vi "Read.vi"(0 "REF IN":refnum<k24>, 1 "error in":errorcluster, 2 "Path":path, 3 "Begin":bool, 4 "stop":bool, 5 "stop 2":bool, 9 "V":dbl, 11 "A":dbl) -> (14 "new reference 2":refnum<k24>, 15 "error out":errorcluster, 16 "String":string)   [LabVIEW 2017]
uses:
  C:/KMotion434/KMotion/Release/KMotion_dotNet.dll
panel:
  out "lines":string[](array[string])
  out "element":dbl
  out "Status Check Done":dbl format="%11.1f"
  out "Numeric":dbl
  out "Array":string[](array[string])
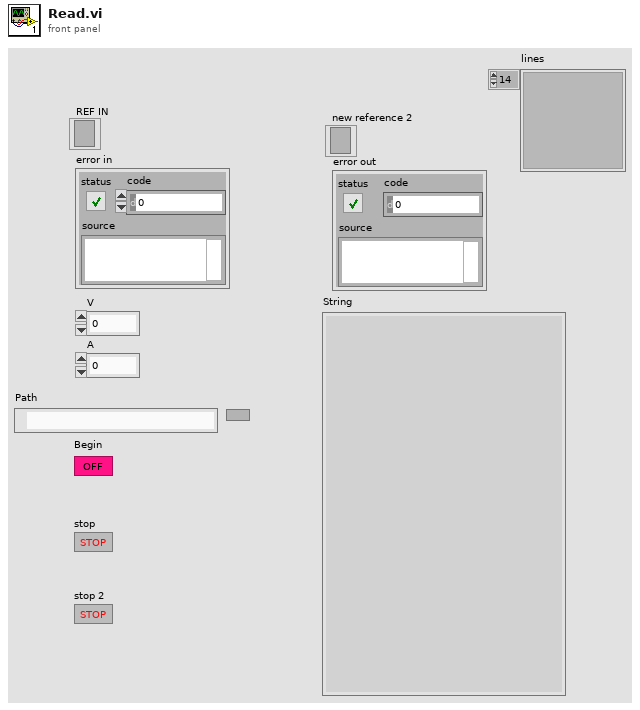
[diagram p1: front panel]
types:
  T1 = cluster{"[0]":dbl, "[1]":dbl, "[2]":dbl, "[3]":dbl, "[4]":dbl, "[5]":dbl, "[6]":dbl, "[7]":dbl, "[8]":dbl, "[9]":dbl, "[10]":dbl, "[11]":dbl}
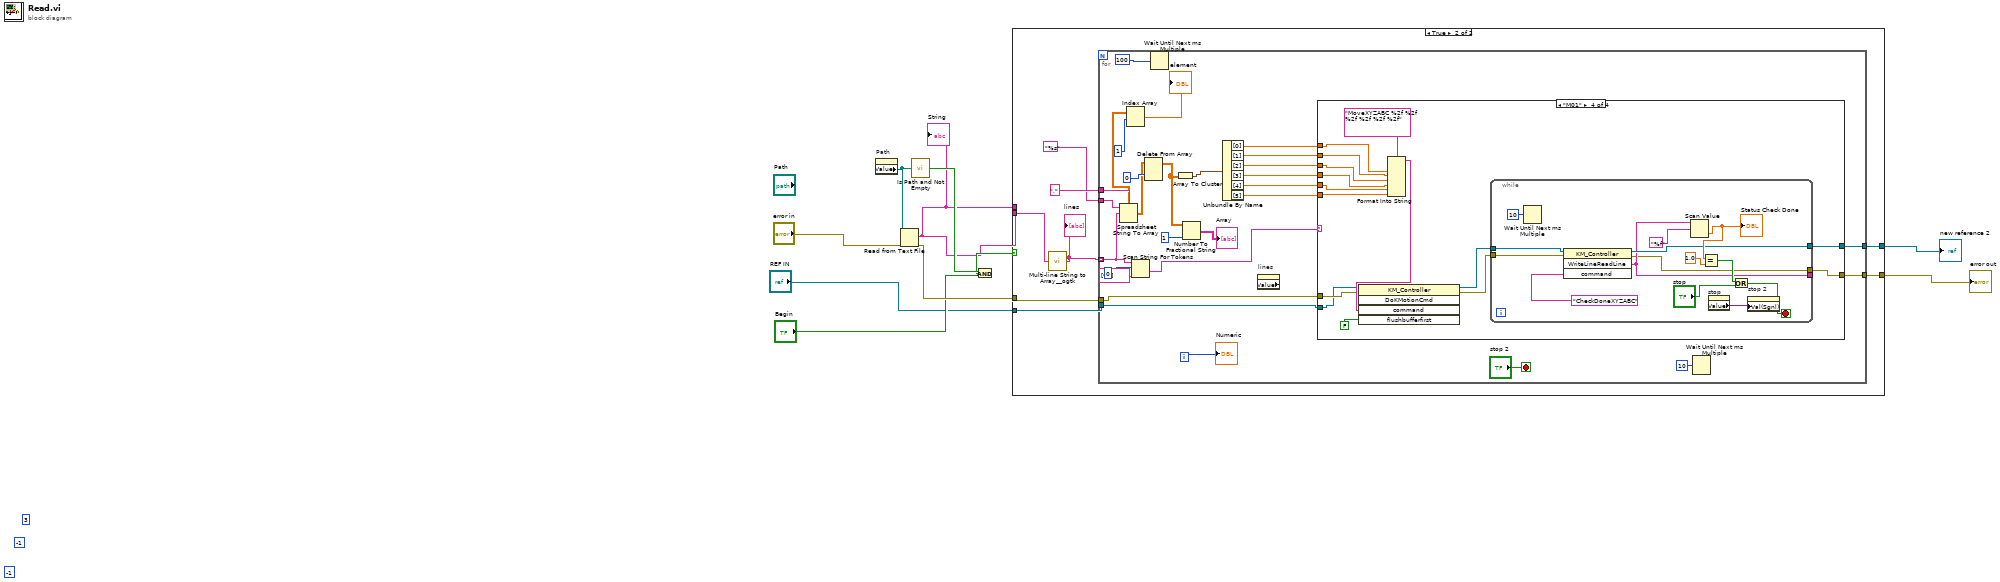
[diagram p0: block diagram]
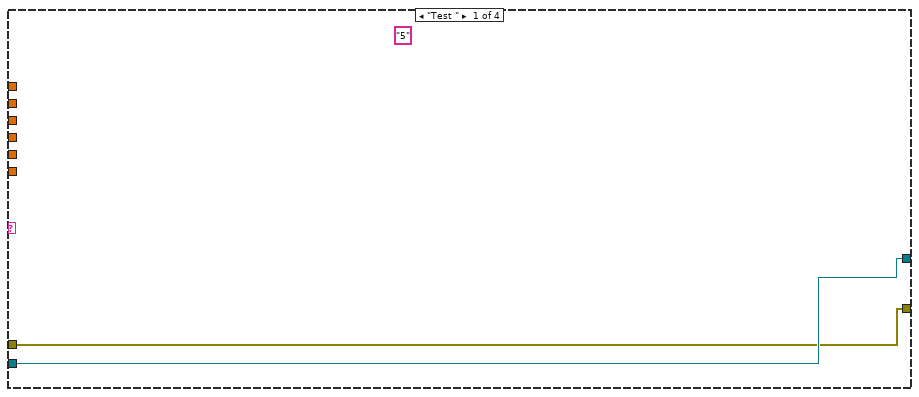
[diagram p3: hidden frame]
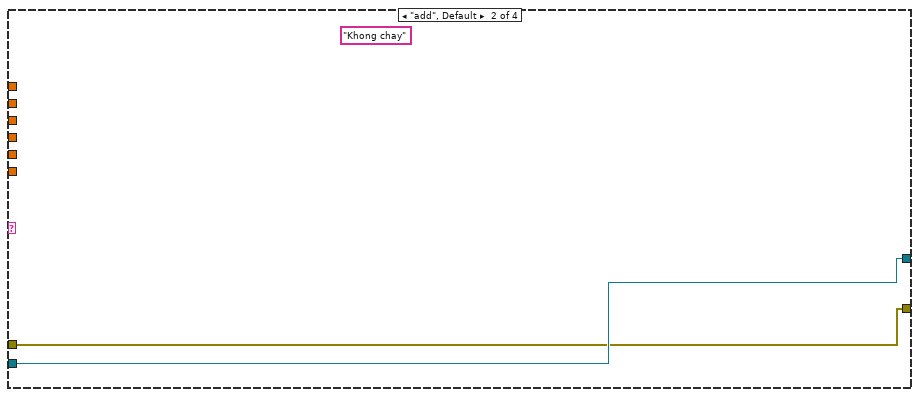
[diagram p4: hidden frame]
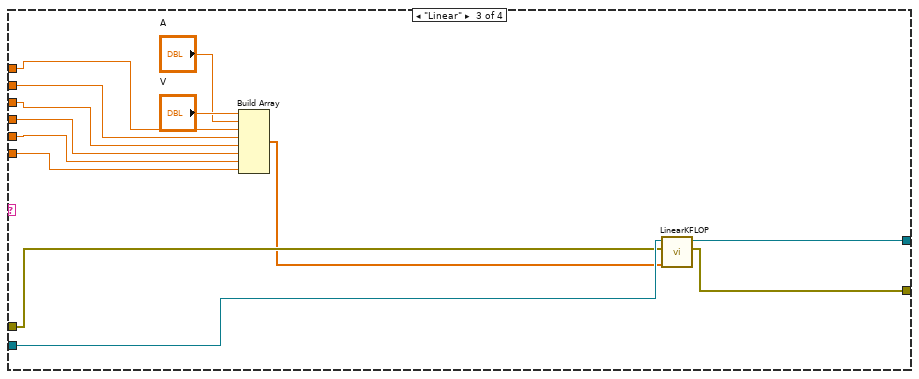
[diagram p5: hidden frame]
diagram:
  (unwired) -1 ("c")
  (unwired) -1 ("b")
  (unwired) 3 ("a")
  n1 = property on="Path" class="Path"() -> ("Value"=w9:path)  [unwired: 2 in, 2 out]
  n2 = Read from Text File(file (use dialog)=w9, error in="error in") -> (text=w1:string, error out=w10:errorcluster)  [unwired: 2 in, 2 out]
  "String" <- w1
  n3 = call <vilib>:"Is Path and Not Empty.vi"("path"=w9) -> ("Is Path and Not Empty?"=w7:bool)  [unwired: 4 in]
  n4 = And(x=w7, y="Begin") -> (x .and. y?=w6:bool)
  n5 = case shown="True" w6 {
    tunnel: "REF IN" -> [w12 w20]
    tunnel: w10 -> [w11 w19]
    tunnel: w1 -> [_ w15]
    tunnel: [w12 w18] -> w3
    tunnel: [w11 w17] -> w2
    tunnel: w1 -> [_ _]
    frame False {
    }
    frame True {
      n6 = call "Multi-line String to Array__ogtk.vi"("string"=w15) -> ("lines"=w16:string[])
      "lines" <- w16
      n7 = for {
        tunnel: w20 -> [w29]
        tunnel: w16 -> [w21] mode=indexing
        tunnel: w19 -> [w28]
        tunnel: [w27] -> w18
        tunnel: [w26] -> w17
        tunnel: "," ("delimiter (Tab)") -> [w24]
        tunnel: "%s" ("format string") -> [w23]
        i -> [w47]
        stop <- "stop 2" stop-if-true
        n8 = Spreadsheet String To Array(delimiter (Tab)=w24, format string=w23, spreadsheet string=w21) -> (array=w22:dbl[][])  [unwired: 1 in]
        n9 = Index Array "Index Array"(array=w22, index (row)=1 ("index")) -> (element=→"element":dbl[])  [unwired: 1 in]
        n10 = Scan String For Tokens(6:string[] [","] ("delimiters (\\s,\\t,\\r,\\n)"), 8:0 ("length (rest)"), 9:w21) -> (1:w37:string)  [unwired: 3 in, 3 out]
        n11 = Delete From Array(array=w22, index (row)=0 ("index")) -> (array with subset deleted=w38:dbl[][])  [unwired: 2 in, 1 out]
        n12 = Wait Until Next ms Multiple(millisecond multiple=u32 100 ("millisecond timer value")) -> ()  [unwired: 1 out]
        n13 = Array To Cluster(array=w38) -> (cluster=w30:T1)
        n14 = Number To Fractional String(number=w38, precision (6)=i16 1) -> (F-format string=→"Array":string[][])  [unwired: 2 in]
        n15 = Unbundle By Name(w30) -> ("[0]"=w36:dbl, "[1]"=w35:dbl, "[2]"=w34:dbl, "[3]"=w33:dbl, "[4]"=w32:dbl, "[5]"=w31:dbl)
        n16 = property on="lines" class="Arr (strict)" props=["Value"]() -> ()  [unwired: 2 in, 3 out]
        n17 = case shown="\"M01\"" w37 {
          tunnel: w36 -> [_ _ w62 w78]
          tunnel: w35 -> [_ _ w61 w77]
          tunnel: w34 -> [_ _ w60 w76]
          tunnel: w33 -> [_ _ w59 w75]
          tunnel: w32 -> [_ _ w58 w74]
          tunnel: w31 -> [_ _ w57 w73]
          tunnel: w29 -> [w50 w52 w65 w68]
          tunnel: w28 -> [w49 w51 w64 w70]
          tunnel: [w50 w52 w54 w67] -> w27
          tunnel: [w49 w51 w53 w66] -> w26
          frame "Test " {
            (unwired) "5"
          }
          frame "add", Default {
            (unwired) "Khong chay"
          }
          frame "Linear" {
            n18 = Build Array("V", "A", w62, w61, w60, w59, w58, w57) -> (w63:dbl[])
            n19 = call "LinearKFLOP.vi"("Array"=w63, "error in (no error)"=w64, "new reference"=w65) -> ("error out"=w53:errorcluster, "new reference 2"=w54:refnum<k24>)  [unwired: 7 in]
          }
          frame "M01" {
            n20 = Format Into String(format string="MoveXYZABC %2f %2f %2f %2f %2f %2f", w78, w77, w76, w75, w74, w73) -> (resulting string=w71:string)  [unwired: 2 in, 1 out]
            n21 = invoke class="KM_Controller" method="DoKMotionCmd"(reference=w68, error in=w70, "command"=w71, "flushbufferfirst"=FALSE) -> (reference out=w69:refnum<k24>, error out=w72:errorcluster)  [unwired: 1 in, 3 out]
            n22 = while {
              tunnel: w72 -> [w86]
              tunnel: w69 -> [w87]
              tunnel: [w85] -> w67
              tunnel: [w84] -> _
              tunnel: [w83] -> w66
              stop <- w89 stop-if-true
              n23 = Wait Until Next ms Multiple(millisecond multiple=u32 10) -> ()  [unwired: 1 out]
              n24 = invoke class="KM_Controller" method="WriteLineReadLine"(reference=w87, error in=w86, "command"="CheckDoneXYZABC") -> (reference out=w85:refnum<k24>, error out=w83:errorcluster, "WriteLineReadLine"=w84:string)  [unwired: 1 in, 1 out]
              n25 = Scan Value(string=w84, format string="%f") -> (value=w92:dbl)  [unwired: 1 in, 1 out]
              "Status Check Done" <- w92
              n26 = Equal?(x=w92, y=1.0 ("x")) -> (x = y?=w88:bool)
              n27 = property on="stop" class="Bool"() -> ("Value"=w81:variant)  [unwired: 2 in, 2 out]
              n28 = Or(x=w88, y="stop") -> (x .or. y?=w89:bool)
              n29 = property on="stop 2" class="Bool"("Val(Sgnl)"=w81) -> ()  [unwired: 2 in, 2 out]
            }
          }
        }
        n30 = Wait Until Next ms Multiple(millisecond multiple=u32 10) -> ()  [unwired: 1 out]
        "Numeric" <- w47
      }
    }
  }
  "new reference 2" <- w3
  "error out" <- w2
